vi "I2C Read 1.vi"(8 "Error in":errorcluster, 9 "size (0)":u32, 10 "Channel":u32 max=5 step=1, 11 "VISA":refnum<visa-resource-name>="COM6") -> (3 "Data Out":u8[](array[numeric]) format="%.0x")   [LabVIEW 2011]
uses:
  <vilib>/Instr/_visa.llb/VISA Configure Serial Port (Instr).vi
panel:
  # "I2C EEPROM Read"
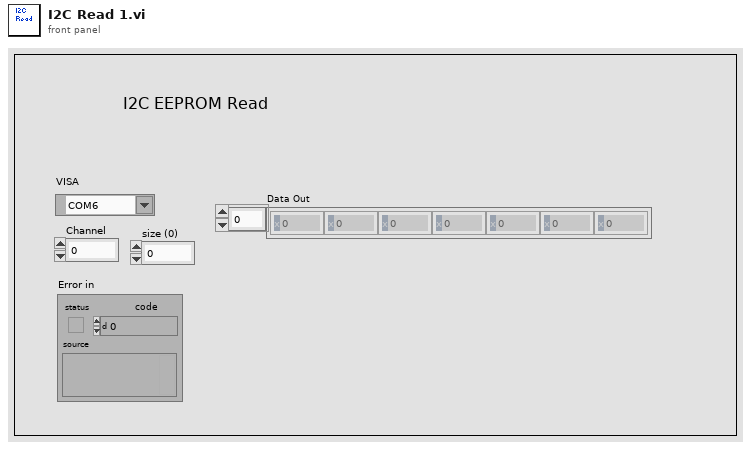
[diagram p1: front panel]
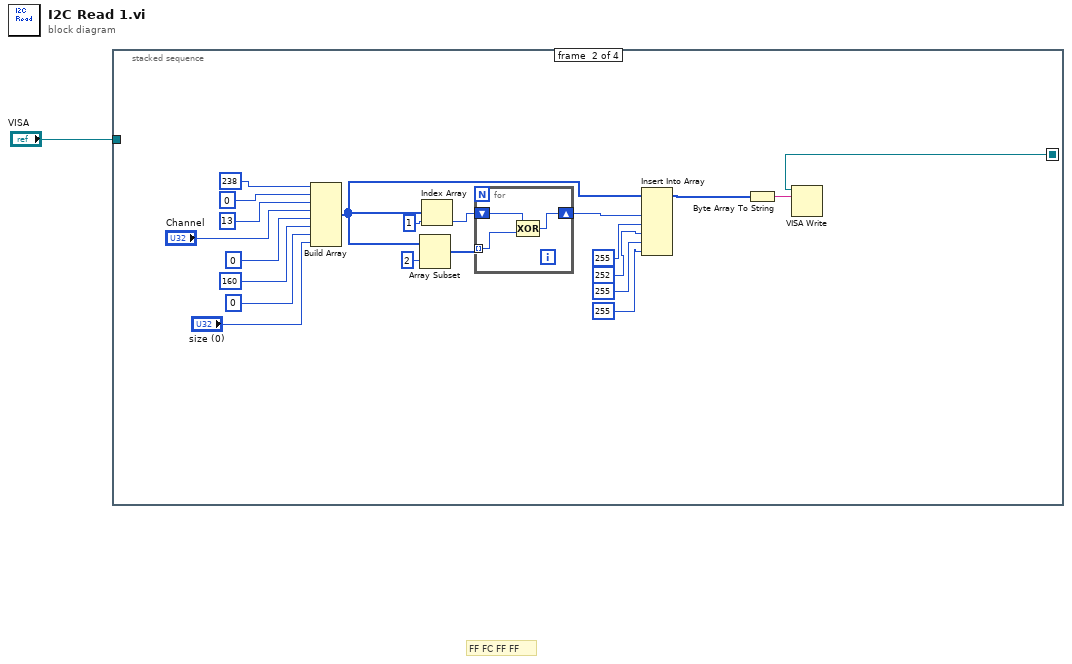
[diagram p0: block diagram]
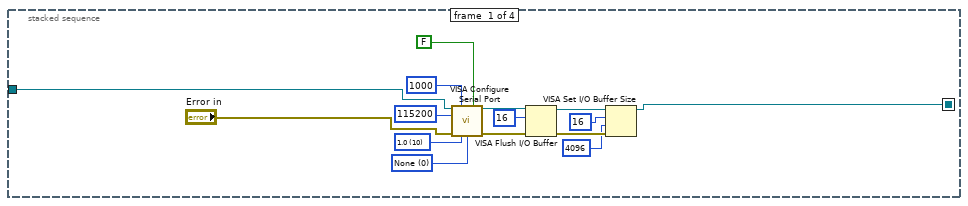
[diagram p2: hidden frame]
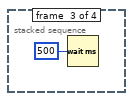
[diagram p3: hidden frame]
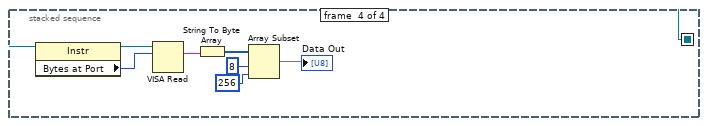
[diagram p4: hidden frame]
diagram:
  # "FF FC FF FF"
  n1 = stacked-sequence {
    seq-local: [w3 _ _ _] -> [_ w17 _ w48]
    tunnel: "VISA" -> [w2 _ _ _]
    frame #0 {
      w15 = u16 0 items=["None", "XON/XOFF", "RTS/CTS", "XON/XOFF & RTS/CTS", "DTR/DSR", "XON/XOFF & DTR/DSR"] ("flow control (0:none)")
      w9 = u16 10 items=["1.0"=10, "1.5"=15, "2.0"=20] ("stop bits (10: 1 bit)")
      n2 = call-poly "VISA Configure Serial Port"("VISA resource name"=w2, "timeout (10sec)"=u32 1000 ("timeout"), "Enable Termination\nChar (T)"=FALSE ("Enable Termination\nChar (T)"), "baud rate (9600)"=u32 115200 ("baud rate"), "error in (no error)"="Error in", "stop bits (10: 1 bit)"=w9, "flow control (0:none)"=w15) -> ("VISA resource name out"=w16:refnum<visa-resource-name>, "error out"=w5:errorcluster)  [unwired: 7 in]
      n3 = VISA Flush I/O Buffer(VISA resource name=w16, mask (16)=u16 16, error in (no error)=w5) -> (VISA resource name out=w12:refnum<visa-resource-name>, error out=w11:errorcluster)
      n4 = VISA Set I/O Buffer Size(VISA resource name=w12, mask (16)=u16 16, size (4096)=u32 4096 ("size (0)"), error in (no error)=w11) -> (VISA resource name out=w3:refnum<visa-resource-name>)  [unwired: 1 out]
    }
    frame #1 {
      n5 = Build Array(u32 238 ("size (0)"), u32 0 ("size (0)"), u32 13 ("size (0)"), "Channel", u32 0 ("size (0)"), u32 160 ("size (0)"), u32 0 ("size (0)"), "size (0)") -> (w25:u32[])
      n6 = Array Subset(array=w25, index=2 ("索引")) -> (w29:u32[])  [unwired: 1 in]
      n7 = Index Array(array=w25, index=1 ("索引")) -> (element=w27:u32)
      n8 = for {
        shift-right: [w38] -> w23
        shift-left: w27 -> [w40]
        tunnel: w29 -> [w39] mode=indexing
        n9 = Compound Arithmetic op=XOR(w40, w39) -> (w38:u32)
      }
      n10 = Insert Into Array(array=w25, new element #1=w23, new element #2=u32 255 ("size (0)"), new element #3=u32 252 ("size (0)"), new element #4=u32 255 ("size (0)"), new element #5=u32 255 ("size (0)")) -> (w18:u32[])  [unwired: 1 in]
      n11 = Byte Array To String(unsigned byte array=w18) -> (string=w24:string)
      n12 = VISA Write(VISA resource name=w17, write buffer=w24) -> ()  [unwired: 1 in, 3 out]
    }
    frame #2 {
      n13 = Wait (ms)(milliseconds to wait=u32 500 ("等待时间（毫秒）")) -> ()  [unwired: 1 out]
    }
    frame #3 {
      n14 = property class="Instr"(reference=w48) -> (reference out=w46:refnum<visa-resource-name>, "Bytes at Port"=w47:u32)  [unwired: 1 in, 1 out]
      n15 = VISA Read(VISA resource name=w46, byte count=w47) -> (read buffer=w49:string)  [unwired: 1 in, 3 out]
      n16 = String To Byte Array(string=w49) -> (unsigned byte array=w45:u8[])
      n17 = Array Subset(array=w45, index=8 ("索引"), length=256 ("长度")) -> (→"Data Out":u8[])
    }
  }
